vi "save_image.vi"(8 "error in (no error)":errorcluster, 9 "dset_name":string="image", 10 "picture":picture, 11 "HDF5 Ref":T1) -> (0 "error out":errorcluster, 3 "HDF5 Ref out":T1)   [LabVIEW 2019]
uses:
  <vilib>/UPVI/lvhdf5/library.llb/HDF5 Ref.ctl
  <vilib>/UPVI/lvhdf5/hdf5_hl.dll
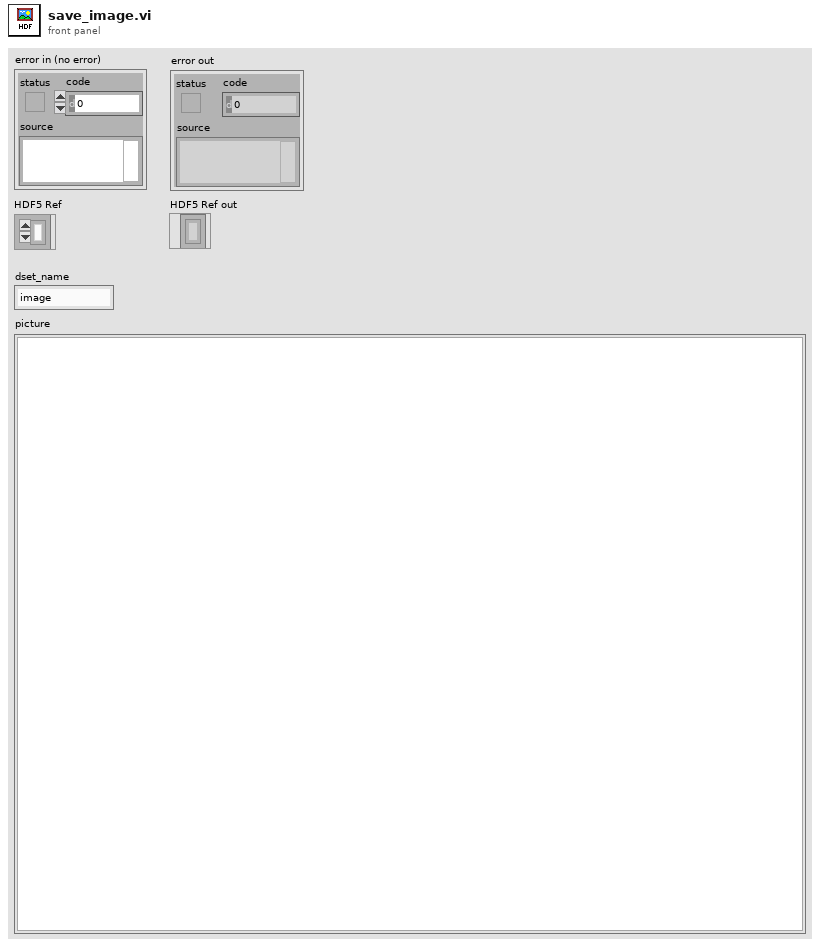
[diagram p1: front panel]
types:
  T1 = typedef "HDF5 Ref.ctl" = refnum<k1>
  T2 = typedef "imagedata.ctl" = cluster{"image type":i32, "image depth":i32, "image":u8[], "mask":u8[], "colors":u32[], "Rectangle":cluster{"left":i16, "top":i16, "right":i16, "bottom":i16}}
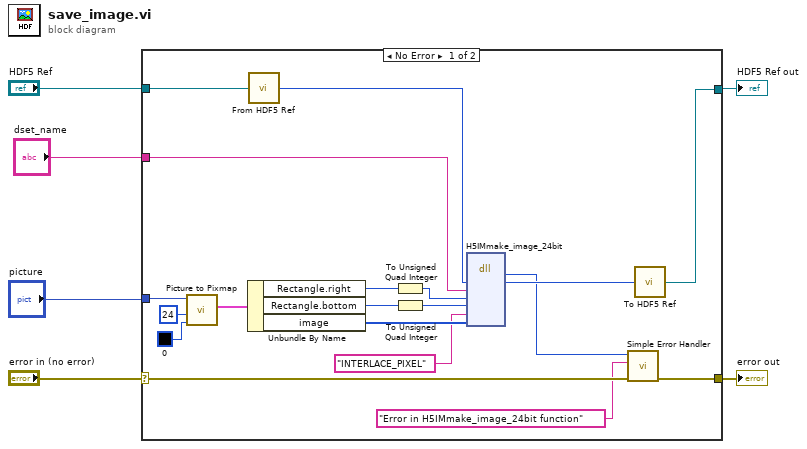
[diagram p0: block diagram]
diagram:
  n1 = case shown="No Error" "error in (no error)" {
    selector: "error in (no error)" -> [w10 w27]
    tunnel: [w14 w26] -> w6
    tunnel: [w11 w27] -> w4
    tunnel: "HDF5 Ref" -> [w13 w26]
    tunnel: "picture" -> [w12 _]
    tunnel: "dset_name" -> [w7 _]
    frame No Error {
      n2 = call <vilib>:"Picture to Pixmap.vi"("Background Color"=u32 0, "depth"=24, "picture"=w12) -> ("image data"=w17:T2)  [unwired: 7 in, 1 out]
      n3 = Unbundle By Name(w17) -> ("Rectangle.right"=w20:i16, "Rectangle.bottom"=w22:i16, "image"=w25:u8[])
      n4 = call <vilib>:"From HDF5 Ref.vi"("HDF5 Ref"=w13) -> ("I32"=w16:i32)
      n5 = To Unsigned Quad Integer(1:w20) -> (0:w21:u64)
      n6 = To Unsigned Quad Integer(1:w22) -> (0:w23:u64)
      n7 = dll-call lib="C:/Program Files/National Instruments/LabVIEW 2019/vi.lib/UPVI/lvhdf5/hdf5_hl.dll" fn="H5IMmake_image_24bit"("loc_id"=w16, "dset_name"=w7, "width"=w21, "height"=w23, "interlace"="INTERLACE_PIXEL", "data"=w25) -> ("return type"=w9:i32, "loc_id"=w15:i32)  [unwired: 8 in, 2 out]
      n8 = call <vilib>:"Simple Error Handler.vi"("error code (no error:0)"=w9, "error source (\" \")"="Error in H5IMmake_image_24bit function" ("error source (\" \")"), "error in (no error)"=w10) -> ("error out"=w11:errorcluster)  [unwired: 2 in, 4 out]
      n9 = call <vilib>:"To HDF5 Ref.vi"("I32"=w15) -> ("HDF5 Ref"=w14:T1)
    }
    frame Error {
    }
  }
  "HDF5 Ref out" <- w6
  "error out" <- w4
